vi "PassObserverRole.vi"(6 "Tactic index in":i32, 9 "first call":bool, 10 "Game in":refnum<class "Game.lvclass">, 11 "PassObserverRole in":refnum<class "PassObserverRole.lvclass">) -> (1 "tactic index":i32, 2 "Robot":refnum<class "Robot.lvclass">, 3 "PassObserverRole out":refnum<class "PassObserverRole.lvclass">)   [LabVIEW 2018, in "PassObserverRole.lvclass"]
uses:
  PassObserverRole.lvclass
  PassObserverTactic_class/PassObserverTactic.lvclass
  Tacticbook_class/Tacticbook.lvclass
  Game_class/Game.lvclass
  Robot_class/Robot.lvclass
panel:
  out "Game out":refnum<class "Game.lvclass">
  out "error out":errorcluster
  in  "error in (no error)":errorcluster
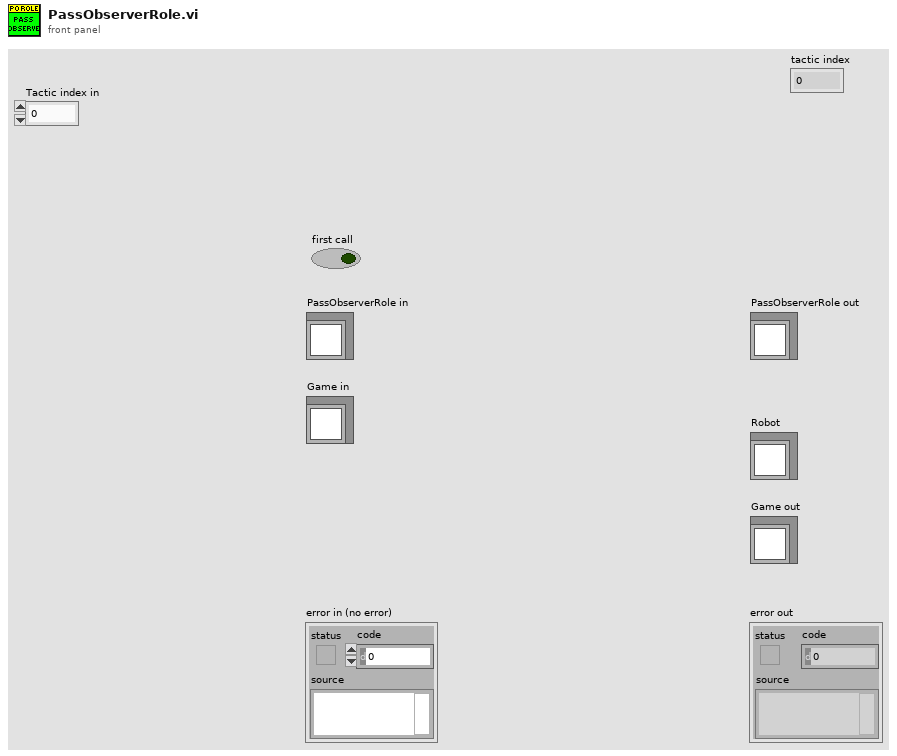
[diagram p1: front panel]
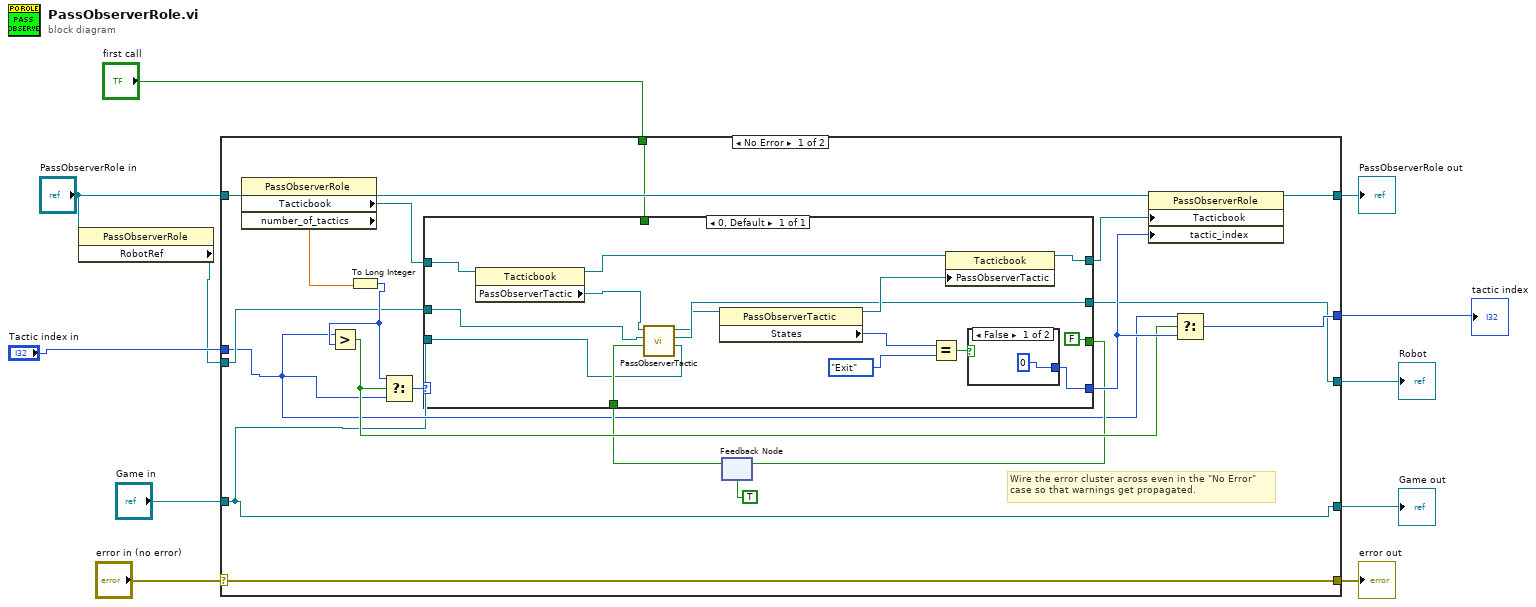
[diagram p0: block diagram]
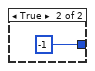
[diagram p2: hidden frame]
diagram:
  n1 = property class="PassObserverRole"(reference="PassObserverRole in") -> ("RobotRef"=w1:refnum<class "Robot.lvclass">)  [unwired: 1 in, 2 out]
  n2 = case shown="No Error" "error in (no error)" {
    selector: "error in (no error)" -> [w31 w53]
    tunnel: [w31 w53] -> w10
    tunnel: [w17 w52] -> w9
    tunnel: "PassObserverRole in" -> [w21 w52]
    tunnel: "Game in" -> [w14 w49]
    tunnel: [w18 w51] -> w7
    tunnel: w1 -> [w20 w51]
    tunnel: [w19 w50] -> w5
    tunnel: "first call" -> [w16 _]
    tunnel: "Tactic index in" -> [w15 w50]
    tunnel: [w14 w49] -> w4
    frame No Error {
      # "Wire the error cluster across even in the \"No Error\"\ncase so that warnings get propagated."
      n3 = property class="PassObserverRole"(reference=w21) -> (reference out=w30:refnum<class "PassObserverRole.lvclass">, "Tacticbook"=w29:refnum<class "Tacticbook.lvclass">, "number_of_tactics"=w13:dbl)  [unwired: 1 in, 1 out]
      n4 = To Long Integer(number=w13) -> (32bit integer=w22:i32)
      n5 = Greater?(x=w15, y=w22) -> (0:w25:bool)
      n6 = Select(t=w22, s=w25, f=w15) -> (s? t:f=w26:i32)
      n7 = feedback #1(TRUE) -> (w23:bool)
      n8 = case shown="0, Default" w26 {
        tunnel: [w40] -> w27
        tunnel: w29 -> [w44]
        tunnel: w20 -> [w37]
        tunnel: [w42] -> w28
        tunnel: w14 -> [w33]
        tunnel: w16 -> [_]
        tunnel: [FALSE] -> w24
        tunnel: w23 -> [w34]
        tunnel: [w36] -> w18
        frame 0, Default {
          n9 = property class="Tacticbook"(reference=w44) -> (reference out=w43:refnum<class "Tacticbook.lvclass">, "PassObserverTactic"=w38:refnum<class "PassObserverTactic.lvclass">)  [unwired: 1 in, 1 out]
          n10 = call-dynamic "PassObserverTactic.vi"("Game in"=w33, "first call"=w34, "Robot"=w37, "PassObserverTactic in"=w38) -> ("Robot"=w36:refnum<class "Robot.lvclass">, "PassObserverTactic out"=w35:refnum<class "PassObserverTactic.lvclass">)  [unwired: 5 in, 1 out]
          n11 = property class="PassObserverTactic"(reference=w35) -> (reference out=w41:refnum<class "PassObserverTactic.lvclass">, "States"=w45:enum16{"PassObserver", "Halt", "Exit"})  [unwired: 1 in, 1 out]
          n12 = Equal?(x=w45, y=enum16{"PassObserver", "Halt", "Exit"}."Exit" ("States")) -> (x = y?=w46:bool)
          n13 = property class="Tacticbook"(reference=w43, "PassObserverTactic"=w41) -> (reference out=w42:refnum<class "Tacticbook.lvclass">)  [unwired: 1 in, 1 out]
          n14 = case shown="False" w46 {
            tunnel: [0 -1] -> w40
            frame False {
            }
            frame True {
            }
          }
        }
      }
      n15 = feedback-in #1(w24) -> ()
      n16 = property class="PassObserverRole"(reference=w30, "Tacticbook"=w28, "tactic_index"=w27) -> (reference out=w17:refnum<class "PassObserverRole.lvclass">)  [unwired: 1 in, 1 out]
      n17 = Select(t=w15, s=w25, f=w27) -> (s? t:f=w19:i32)
    }
    frame Error {
    }
  }
  "error out" <- w10
  "PassObserverRole out" <- w9
  "Game out" <- w4
  "Robot" <- w7
  "tactic index" <- w5
